vi "FGVSteps.vi"(7 "Enum":T1, 8 "error in":errorcluster, 9 "stepsglobalCounterIn":i32, 10 "stepsLeftIn":i32, 11 "stepsIn":i32) -> (0 "error out":errorcluster, 1 "stepglobalCounterOut":i32, 2 "stepsLeftOut":i32, 3 "stepsOut":i32)   [LabVIEW 2016]
uses:
  controls/Enum.ctl
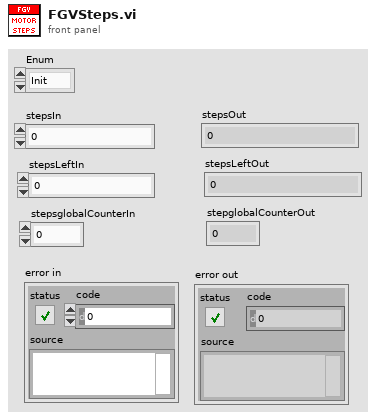
[diagram p1: front panel]
types:
  T1 = typedef "Enum.ctl" = enum16{"Init", "Read", "Write"}
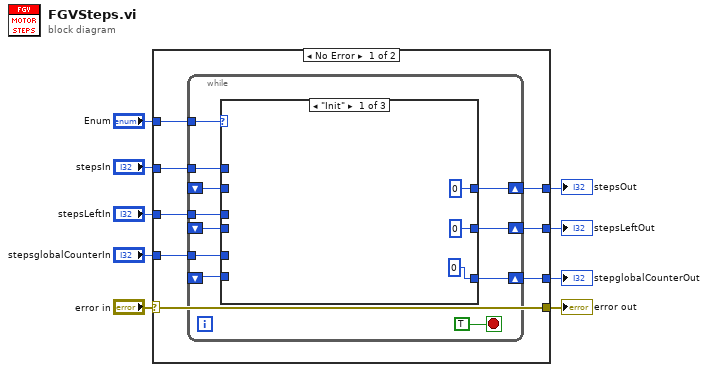
[diagram p0: block diagram]
diagram:
  n1 = case shown="No Error" "error in" {
    selector: "error in" -> [w16 w41]
    tunnel: "Enum" -> [w17 _]
    tunnel: [w16 w41] -> w8
    tunnel: "stepsIn" -> [w15 w40]
    tunnel: [w14 w40] -> w6
    tunnel: "stepsLeftIn" -> [w13 w39]
    tunnel: [w12 w39] -> w3
    tunnel: "stepsglobalCounterIn" -> [w10 w38]
    tunnel: [w11 w38] -> w1
    frame No Error {
      n2 = while {
        tunnel: w17 -> [w27]
        tunnel: w15 -> [w26]
        shift-right: [w25] -> w14
        shift-left: _ -> [w24]
        tunnel: w13 -> [w23]
        shift-right: [w22] -> w12
        shift-left: _ -> [w21]
        shift-right: [w19] -> w11
        shift-left: _ -> [w20]
        tunnel: w10 -> [w18]
        stop <- TRUE stop-if-true
        n3 = case shown="\"Init\"" w27 {
          tunnel: w26 -> [_ _ w37]
          tunnel: [0 ("stepsIn") w34 w37] -> w25
          tunnel: w24 -> [_ w34 _]
          tunnel: w23 -> [_ _ w36]
          tunnel: [0 ("stepsLeftIn") w33 w36] -> w22
          tunnel: w21 -> [_ w33 _]
          tunnel: w20 -> [_ w32 _]
          tunnel: [0 ("stepsLeftIn") w32 w35] -> w19
          tunnel: w18 -> [_ _ w35]
          frame "Init" {
          }
          frame "Read", Default {
          }
          frame "Write" {
          }
        }
      }
    }
    frame Error {
    }
  }
  "error out" <- w8
  "stepsOut" <- w6
  "stepsLeftOut" <- w3
  "stepglobalCounterOut" <- w1
